vi "Connect to Machine .vi"(8 "error in":errorcluster, 9 "Firmware":string(combo), 11 "Machine In":refnum<visa-resource-name>="COM3") -> (0 "error out":errorcluster, 1 "Firmware":string, 3 "Machine Out":refnum<visa-resource-name>)   [LabVIEW 2017]
doc: "Connects to specified device over USB. \n\n<B>Inputs</B>: \n- Machine In: Specifies the desired machine connected to computer via USB.\n- Firmware: Specifies the machine firmware. Supported firmwares are Grbl and uArm Swift Pro.\n\n<B>Outputs</B>: \n- Machine Out: Reference to the selected USB device.\n- Firmware: Specifies the machine firmware.\n- Error Out: returns an error if one occurs in vi (or has occurred in a previous vi), and passes it to next wired terminal."
uses:
  <vilib>/Instr/_visa.llb/VISA Configure Serial Port (Instr).vi
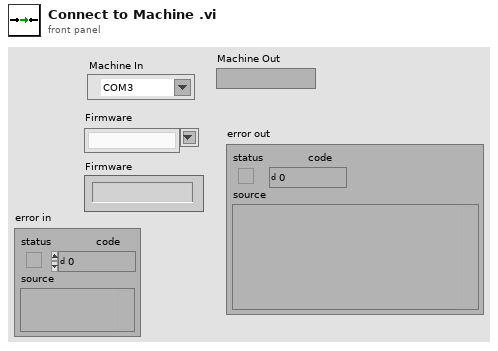
[diagram p1: front panel]
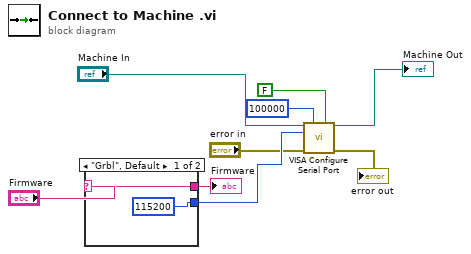
[diagram p0: block diagram]
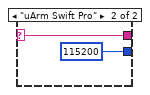
[diagram p2: hidden frame]
diagram:
  n1 = case shown="\"Grbl\", Default" "Firmware" {
    selector: "Firmware" -> [w10 w12]
    tunnel: [115200 u32 115200 ("baud rate (9600)")] -> w3
    tunnel: [w10 w12] -> w2
    frame "Grbl", Default {
    }
    frame "uArm Swift Pro" {
    }
  }
  "Firmware" <- w2
  n2 = call-poly "VISA Configure Serial Port"("VISA resource name"="Machine In", "timeout (10sec)"=u32 100000, "Enable Termination\nChar (T)"=FALSE ("Enable Termination\nChar (T)"), "baud rate (9600)"=w3, "error in (no error)"="error in") -> ("VISA resource name out"=→"Machine Out":refnum<visa-resource-name>, "error out"=→"error out":errorcluster)  [unwired: 9 in]
